vi "Data Load.vi"(0 "VISA Resource Name":refnum<visa-resource-name>, 1 "Upload Data (0)":i16[](array[numeric]), 5 "Action (T:UPLOAD)":bool=TRUE, 9 "File Name (USER_DATA)":string="USER_DATA", 11 "error in (no error)":errorcluster {"code" format="%.0x"}) -> (4 "VISA Resource Name Out":refnum<visa-resource-name>, 6 "Download Data":i16[](array[numeric]), 15 "error out":errorcluster {"code" format="%.0x"})   [LabVIEW 2012, in "Agilent ESG Series.lvlib"]
doc: "This VI is used to upload or download a block of data to or from the specified memory location (filename)."
uses:
  <instrlib>/Agilent ESG Series/Agilent ESG Series.lvlib
panel:
  # "UPLOAD"
  # "DOWNLOAD"
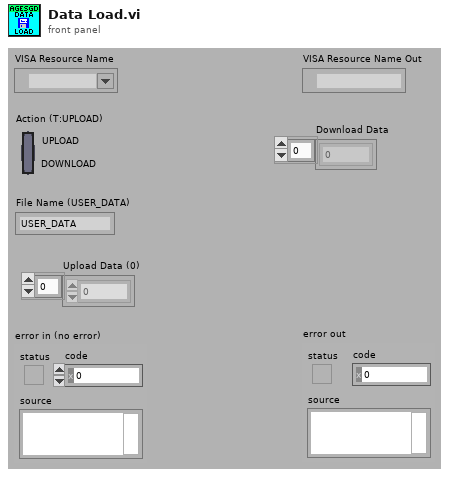
[diagram p1: front panel]
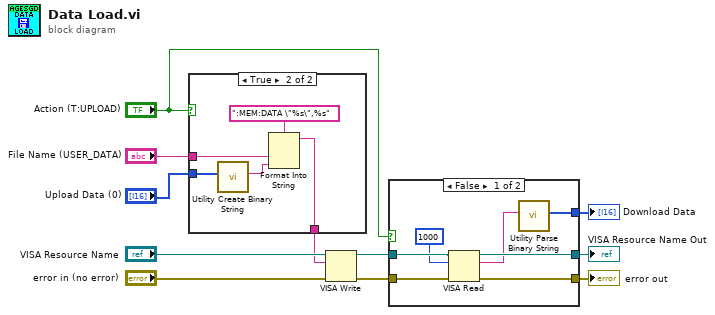
[diagram p0: block diagram]
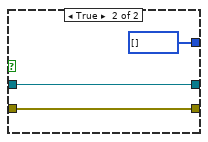
[diagram p2: hidden frame]
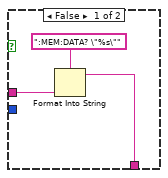
[diagram p3: hidden frame]
diagram:
  n1 = case shown="True" "Action (T:UPLOAD)" {
    tunnel: "Upload Data (0)" -> [_ w16]
    tunnel: "File Name (USER_DATA)" -> [w13 w18]
    tunnel: [w12 w17] -> w9
    frame False {
      n2 = Format Into String(format string=":MEM:DATA? \"%s\"", w13) -> (resulting string=w12:string)  [unwired: 2 in, 1 out]
    }
    frame True {
      n3 = call <instrlib>:"Utility Create Binary String.vi"("Input Array"=w16) -> ("Binary String"=w15:string)  [unwired: 10 in]
      n4 = Format Into String(format string=":MEM:DATA \"%s\",%s", w18, w15) -> (resulting string=w17:string)  [unwired: 2 in, 1 out]
    }
  }
  n5 = VISA Write(VISA resource name="VISA Resource Name", write buffer=w9, error in (no error)="error in (no error)") -> (VISA resource name out=w5:refnum<visa-resource-name>, error out=w4:errorcluster)  [unwired: 1 out]
  n6 = case shown="False" "Action (T:UPLOAD)" {
    tunnel: w5 -> [w26 w29]
    tunnel: w4 -> [w25 w28]
    tunnel: [w24 w28] -> w3
    tunnel: [w23 w29] -> w2
    tunnel: [w20 i32[] []] -> w1
    frame False {
      n7 = VISA Read(VISA resource name=w26, byte count=u32 1000 ("byte count (0)"), error in (no error)=w25) -> (VISA resource name out=w23:refnum<visa-resource-name>, read buffer=w21:string, error out=w24:errorcluster)  [unwired: 1 out]
      n8 = call <instrlib>:"Utility Parse Binary String.vi"("Input Binary String"=w21) -> ("Output Array"=w20:i16[])  [unwired: 10 in]
    }
    frame True {
    }
  }
  "error out" <- w3
  "VISA Resource Name Out" <- w2
  "Download Data" <- w1
